vi "Molar Mass of Humid Air (Kg to Mol).vi"(1 "Gas Presure":dbl[unit]=80000.0 min=80000.0 max=120000.0, 2 "Tceg":dbl[unit], 3 "RH":dbl) -> (0 "MMH\nMolar Mass of Humid Air (Kg/mol)":dbl[unit])   [LabVIEW 2018]
panel:
  out "M-W":dbl[unit]=0.018
  out "MMH\nMolar Mass of Humid Air (Kg/mol)":dbl[unit](knob) scale=0.0..0.05
  out "M-da 3":dbl[unit]=0.029
  out "Temprature Of Input Air\nKelvin Degree":dbl[unit](slide) scale=273.0..373.0
  out "Tk":dbl[unit]
  out "Temprature Of Input Air\nCentigrade Degree":dbl[unit](slide) scale=0.0..100.0
  out "Humidity of Input Air":dbl(knob) scale=0.0..100.0
  out "R":dbl[unit]
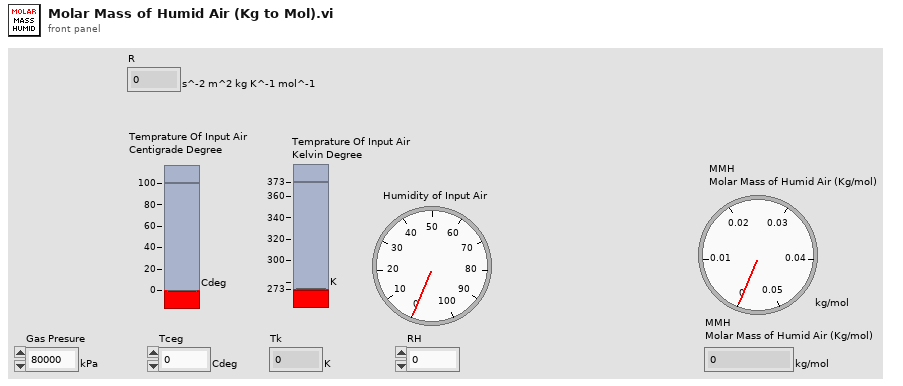
[diagram p1: front panel]
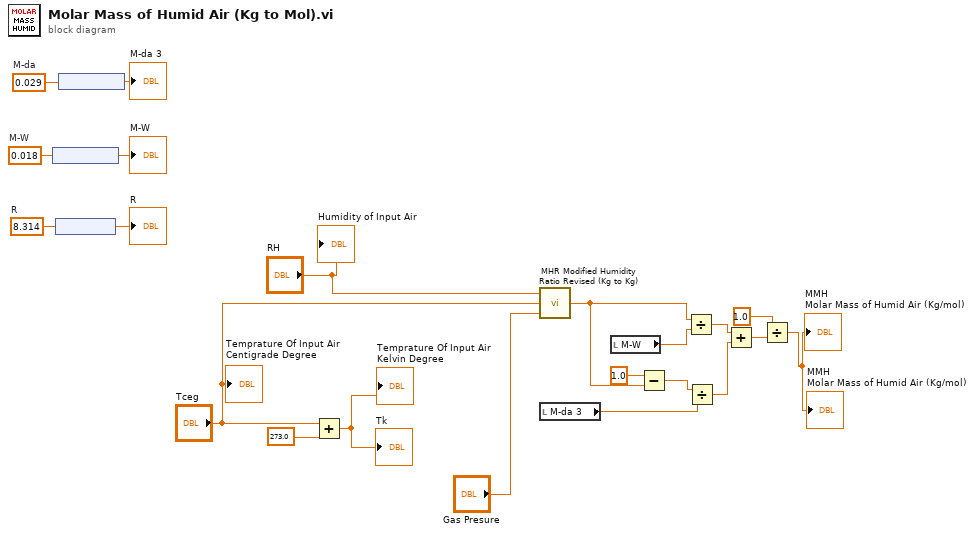
[diagram p0: block diagram]
diagram:
  w11 = 0.018  # M-W
  w9 = 0.029  # M-da
  w21 = 8.314  # R
  n1 = node(w11) -> (→"M-W":dbl[unit])
  n2 = node(w21) -> (→"R":dbl[unit])
  n3 = node(w9) -> (→"M-da 3":dbl[unit])
  n4 = Add(x="Tceg", y=dbl[unit] 273.0) -> (x+y=→"Tk" →"Temprature Of Input Air\nKelvin Degree":dbl[unit])
  n5 = call "MHR Modified Humidity Ratio Revised (Kg to Kg).vi"("Gas Presure"="Gas Presure", "Tceg"="Tceg", "RH"="RH") -> ("MHR\nModified Humidity Ratio"=w4:dbl)
  n6 = local read "M-da 3"() -> (w6:dbl[unit])
  n7 = local read "M-W"() -> (w5:dbl[unit])
  n8 = Subtract(x=1.0, y=w4) -> (x-y=w13:dbl)
  n9 = Divide(x=w4, y=w5) -> (x/y=w16:dbl[unit])
  n10 = Divide(x=w13, y=w6) -> (x/y=w15:dbl[unit])
  n11 = Add(x=w16, y=w15) -> (x+y=w17:dbl[unit])
  n12 = Divide(x=1.0, y=w17) -> (x/y=→"MMH\nMolar Mass of Humid Air (Kg/mol)" →"MMH\nMolar Mass of Humid Air (Kg/mol)":dbl[unit])
  "Humidity of Input Air" <- "RH"
  "Temprature Of Input Air\nCentigrade Degree" <- "Tceg"
